vi "Run.vi"(7 "Team Index":i32, 8 "Column":i32, 9 "Row":i32, 10 "View":i32[](array[numeric]) caption="View (Team Index, -1: empty)", 11 "third In":refnum<class "third.lvclass">) -> (0 "Replicated":refnum<class "Square.lvclass">, 1 "Direction":T1, 2 "Action":T2, 3 "Square Out":refnum<class "Square.lvclass">)   [LabVIEW 2015, in "third.lvclass"]
uses:
  third.lvclass
  Square/Square.lvclass
  Type Defs/Action Enum.ctl
  Type Defs/Direction Enum.ctl
  third.lvclass/third.ctl
  Common/personality.ctl
  data/Write Direction.vi
  data/Write move count.vi
  data/Write Lifetime.vi
  data/Write Personality.vi
  data/Write Replicated.vi
  data/Write Initialized.vi
  data/Read Replicated.vi
  data/Read Lifetime.vi
  data/Read Personality.vi
  data/Read move count.vi
  data/Read Direction.vi
  data/Read Initialized.vi
  SubVIs/Read-Only Globals.vi
  SubVIs/Globals (private).vi
  variables/trend.vi
  Common/JFD_Common.lvlib
  Type Defs/SB Type Defs.lvlib
panel:
  in  "error in (no error)":errorcluster
  out "error out":errorcluster
  # "NW\nN\nNE\nE\nSE\nS\nSW\nW"
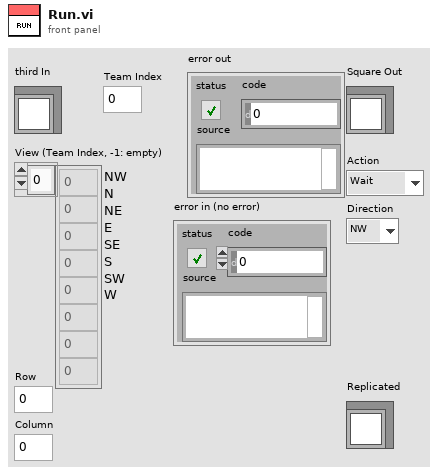
[diagram p1: front panel]
types:
  T1 = typedef "SB Type Defs.lvlib/Direction Enum.ctl" = enum16{"NW", "N", "NE", "E", "SE", "S", "SW", "W"}
  T2 = typedef "SB Type Defs.lvlib/Action Enum.ctl" = enum16{"Wait", "Move", "Attack", "Replicate"}
  T3 = typedef "JFD_Common.lvlib/personality.ctl" = enum16{"aggressor", "replicator"}
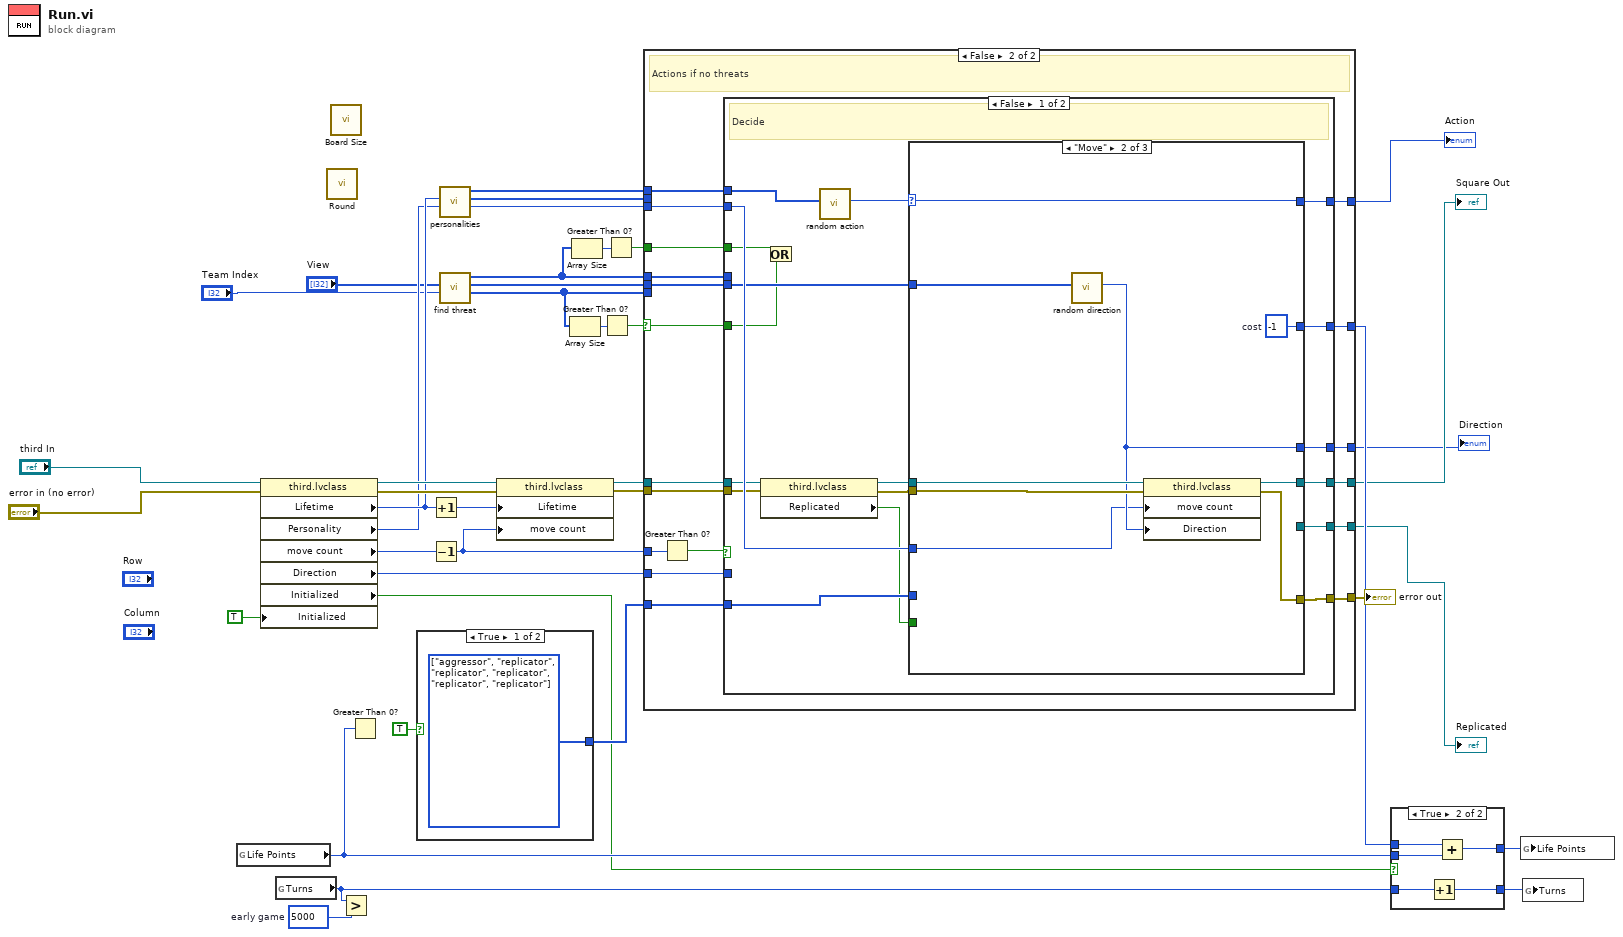
[diagram p0: block diagram]
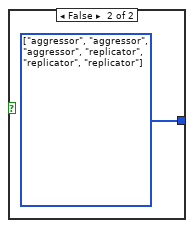
[diagram p2: hidden frame]
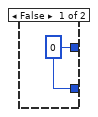
[diagram p3: hidden frame]
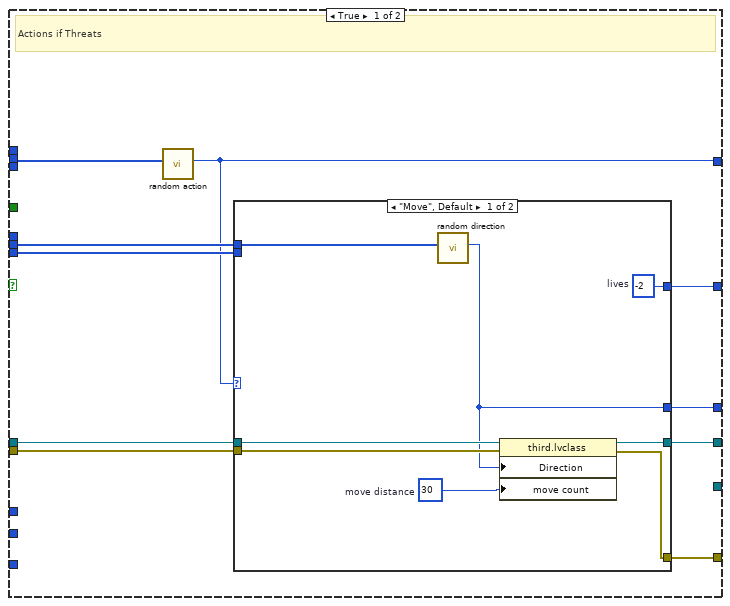
[diagram p4: hidden frame]
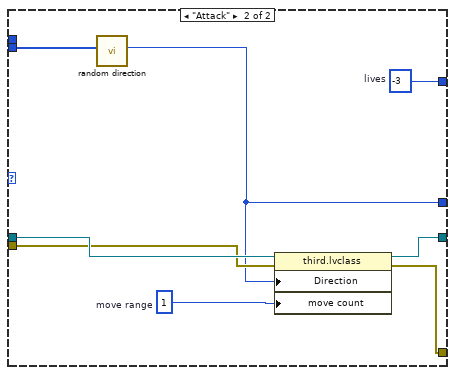
[diagram p5: hidden frame]
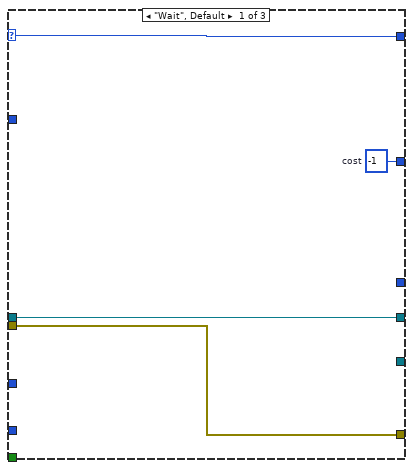
[diagram p6: hidden frame]
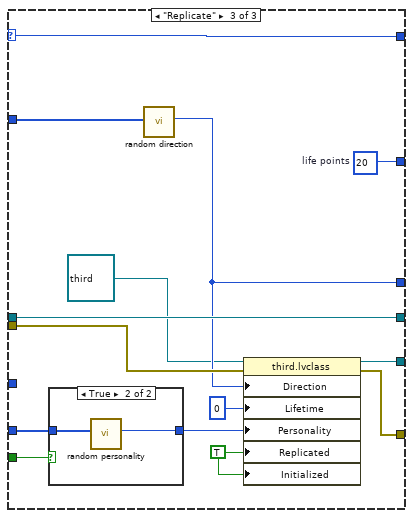
[diagram p7: hidden frame]
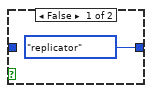
[diagram p8: hidden frame]
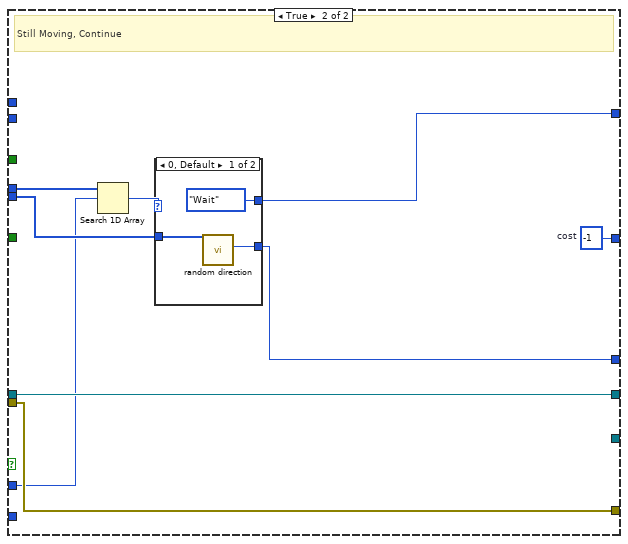
[diagram p9: hidden frame]
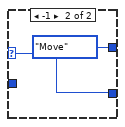
[diagram p10: hidden frame]
diagram:
  w14 = i64 5000  # early game
  n1 = global read "trend.vi" "Life Points"() -> (w19:i64)
  n2 = property class="third.lvclass"(reference="third In", error in="error in (no error)", "Initialized"=TRUE) -> (reference out=w37:refnum<class "third.lvclass">, error out=w38:errorcluster, "Lifetime"=w35:i64, "Personality"=w30:T3, "move count"=w23:i32, "Direction"=w24:T1, "Initialized"=w16:bool)
  n3 = global read "trend.vi" "Turns"() -> (w15:i64)
  n4 = call "Round.vi"() -> ()  [unwired: 11 in, 1 out]
  n5 = call "Board Size.vi"() -> ()  [unwired: 11 in, 1 out]
  n6 = Greater?(x=w15, y=w14) -> ()  [unwired: 1 out]
  n7 = Greater Than 0?(x=w19) -> ()  [unwired: 1 out]
  n8 = case shown="True" TRUE {
    tunnel: [w40 w41] -> w31
    frame True {
      w40 = T3[] [enum."aggressor", enum."replicator", enum."replicator", enum."replicator", enum."replicator", enum."replicator"] items=["aggressor", "replicator"] ("Personalities to choose from")
    }
    frame False {
      w41 = T3[] [enum."aggressor", enum."aggressor", enum."aggressor", enum."replicator", enum."replicator", enum."replicator"] items=["aggressor", "replicator"] ("Personalities to choose from")
    }
  }
  n9 = Increment(x=w35) -> (x+1=w39:i64)
  n10 = Decrement(x=w23) -> (x-1=w22:i32)
  n11 = call "personalities.vi"("Personality"=w30, "Lifetime"=w35) -> ("move"=w32:i32, "threats"=w33:T2[], "no threats"=w34:T2[])  [unwired: 7 in]
  n12 = call "find threat.vi"("Team Index"="Team Index", "View"="View") -> ("Enemy Squares"=w29:T1[], "Empty Squares"=w28:T1[], "Friendly Squares"=w3:T1[])  [unwired: 7 in]
  n13 = property class="third.lvclass"(reference=w37, error in=w38, "Lifetime"=w39, "move count"=w22) -> (reference out=w36:refnum<class "third.lvclass">, error out=w25:errorcluster)
  n14 = Array Size(array=w29) -> (size(s)=w27:i32)
  n15 = Array Size(array=w3) -> (size(s)=w2:i32)
  n16 = Greater Than 0?(x=w27) -> (x > 0?=w26:bool)
  n17 = Greater Than 0?(x=w2) -> (x > 0?=w1:bool)
  n18 = case shown="False" w26 {
    selector: w26 -> [_ w68]
    tunnel: w36 -> [w48 w81]
    tunnel: w25 -> [w49 w85]
    tunnel: [w47 w80] -> w12
    tunnel: [w50 w83] -> w8
    tunnel: [w43 w78] -> w10
    tunnel: [w51 w84] -> w11
    tunnel: [_ w79] -> w13
    tunnel: w32 -> [_ w82]
    tunnel: w34 -> [_ w76]
    tunnel: w33 -> [w46 _]
    tunnel: w31 -> [_ w77]
    tunnel: w29 -> [w45 _]
    tunnel: w28 -> [w44 w75]
    tunnel: w22 -> [_ w74]
    tunnel: w24 -> [_ w72]
    tunnel: w3 -> [_ w71]
    tunnel: [w42 w70] -> w20
    tunnel: w1 -> [_ w69]
    frame True {
      # "Actions if Threats"
      n19 = call "random action.vi"("Actions to choose from"=w46) -> ("Action"=w43:T2)  [unwired: 10 in]
      n20 = case shown="\"Move\", Default" w43 {
        tunnel: [w53 w61] -> w51
        tunnel: w48 -> [w59 w67]
        tunnel: [w58 w66] -> w47
        tunnel: [w57 w65] -> w50
        tunnel: w49 -> [w56 w64]
        tunnel: w45 -> [_ w62]
        tunnel: w44 -> [w54 _]
        tunnel: [w52 w60] -> w42
        frame "Move", Default {
          w52 = i64 -2  # lives
          w55 = 30  # move distance
          n21 = call "random direction.vi"("Directions to Choose From"=w54) -> ("Direction"=w53:T1)  [unwired: 10 in]
          n22 = property class="third.lvclass"(reference=w59, error in=w56, "Direction"=w53, "move count"=w55) -> (reference out=w58:refnum<class "third.lvclass">, error out=w57:errorcluster)
        }
        frame "Attack" {
          w60 = i64 -3  # lives
          w63 = 1  # move range
          n23 = call "random direction.vi"("Directions to Choose From"=w62) -> ("Direction"=w61:T1)  [unwired: 10 in]
          n24 = property class="third.lvclass"(reference=w67, error in=w64, "Direction"=w61, "move count"=w63) -> (reference out=w66:refnum<class "third.lvclass">, error out=w65:errorcluster)
        }
      }
    }
    frame False {
      # "Actions if no threats"
      n25 = Greater Than 0?(x=w74) -> (x > 0?=w73:bool)
      n26 = case shown="False" w73 {
        tunnel: w85 -> [w88 w141]
        tunnel: [w103 w140] -> w84
        tunnel: [w102 w141] -> w83
        tunnel: w82 -> [w101 _]
        tunnel: w81 -> [w100 w142]
        tunnel: [w99 w142] -> w80
        tunnel: [w98 _] -> w79
        tunnel: [w97 w134] -> w78
        tunnel: w77 -> [w96 _]
        tunnel: w76 -> [w94 _]
        tunnel: w75 -> [w95 w139]
        tunnel: w72 -> [_ w136]
        tunnel: w71 -> [_ w137]
        tunnel: [w92 w138] -> w70
        tunnel: w69 -> [w87 _]
        tunnel: w68 -> [w86 _]
        frame False {
          # "Decide"
          n27 = property class="third.lvclass"(reference=w100, error in=w88) -> (reference out=w91:refnum<class "third.lvclass">, error out=w89:errorcluster, "Replicated"=w90:bool)
          n28 = Or(x=w87, y=w86) -> ()  [unwired: 1 out]
          n29 = call "random action.vi"("Actions to choose from"=w94) -> ("Action"=w93:T2)  [unwired: 10 in]
          n30 = case shown="\"Move\"" w93 {
            selector: w93 -> [w105 w112 w122]
            tunnel: [_ w111 w126] -> w103
            tunnel: [w107 w116 w130] -> w102
            tunnel: w89 -> [w107 w115 w129]
            tunnel: w101 -> [_ w108 _]
            tunnel: [w106 w113 w128] -> w99
            tunnel: w91 -> [w106 w114 w128]
            tunnel: [_ _ w127] -> w98
            tunnel: [w105 w112 w122] -> w97
            tunnel: w96 -> [_ _ w124]
            tunnel: w95 -> [_ w110 w121]
            tunnel: [w104 w109 w120] -> w92
            tunnel: w90 -> [_ _ w118]
            frame "Wait", Default {
              w104 = i64 -1  # cost
            }
            frame "Move" {
              w109 = i64 -1  # cost
              n31 = call "random direction.vi"("Directions to Choose From"=w110) -> ("Direction"=w111:T1)  [unwired: 10 in]
              n32 = property class="third.lvclass"(reference=w114, error in=w115, "move count"=w108, "Direction"=w111) -> (reference out=w113:refnum<class "third.lvclass">, error out=w116:errorcluster)
            }
            frame "Replicate" {
              w119 = TRUE ("Replicated")
              w120 = i64 20  # life points
              n33 = case shown="True" w118 {
                tunnel: w124 -> [_ w133]
                tunnel: [personality."replicator" ("Personality") w132] -> w123
                frame False {
                }
                frame True {
                  n34 = call "random personality.vi"("Personalities to choose from"=w133) -> ("Personality"=w132:T3)  [unwired: 10 in]
                }
              }
              n35 = call "random direction.vi"("Directions to Choose From"=w121) -> ("Direction"=w126:T1)  [unwired: 10 in]
              n36 = property class="third.lvclass"(reference=refnum<class "third.lvclass"> refnum ("third.lvclass"), error in=w129, "Direction"=w126, "Lifetime"=i64 0, "Personality"=w123, "Replicated"=w119, "Initialized"=w119) -> (reference out=w127:refnum<class "third.lvclass">, error out=w130:errorcluster)
            }
          }
        }
        frame True {
          w138 = i64 -1  # cost
          # "Still Moving, Continue"
          n37 = Search 1D Array(1D array=w137, element=w136) -> (index of element=w135:i32)  [unwired: 1 in]
          n38 = case shown="0, Default" w135 {
            selector: w135 -> [_ w147]
            tunnel: [w145 w147] -> w140
            tunnel: w139 -> [w144 _]
            tunnel: [Action_Enum."Wait" ("Action") Action_Enum."Move" ("Action")] -> w134
            frame 0, Default {
              n39 = call "random direction.vi"("Directions to Choose From"=w144) -> ("Direction"=w145:T1)  [unwired: 10 in]
            }
            frame -1 {
            }
          }
        }
      }
    }
  }
  "Square Out" <- w12
  "Action" <- w10
  "Direction" <- w11
  "Replicated" <- w13
  "error out" <- w8
  n40 = case shown="True" w16 {
    tunnel: [w148 w153] -> w21
    tunnel: w20 -> [_ w152]
    tunnel: w19 -> [_ w151]
    tunnel: w15 -> [_ w150]
    tunnel: [w148 w149] -> w17
    frame False {
      w148 = i64 0
    }
    frame True {
      n41 = Increment(x=w150) -> (x+1=w149:i64)
      n42 = Add(x=w152, y=w151) -> (x+y=w153:i64)
    }
  }
  n43 = global write "trend.vi" "Life Points"(w21) -> ()
  n44 = global write "trend.vi" "Turns"(w17) -> ()
